vi "check convergence.vi"(4 "number of function evaluations":i32, 6 "current iteration":i32, 7 "stopping criteria":T1={"function tolerance"=1e-06, "parameter tolerance"=1e-06, "max iterations"=0, "max function calls"=0, "gradient tolerance"=0.0, "max time (sec)"=1000.0, "initial tick count"=0}, 9 "gradient":dbl[](array[numeric]), 10 "X":dbl[](array[numeric]), 11 "f":dbl) -> (0 "error out":errorcluster, 1 "xtol":dbl, 2 "ftol":dbl, 3 "stop?":bool, 5 "line search tol":dbl)   [LabVIEW 2017, in "NI_Gmath.lvlib"]
uses:
  <vilib>/gmath/NI_Gmath.lvlib
  <vilib>/gmath/NumericalOptimization/stopping criteria with time.ctl
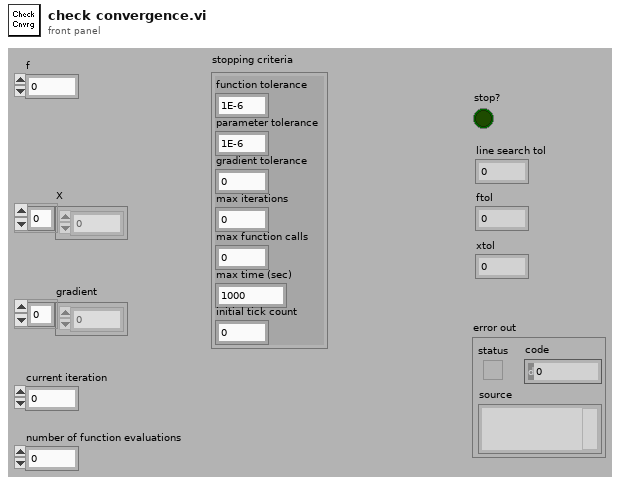
[diagram p1: front panel]
types:
  T1 = typedef "NI_Gmath.lvlib/stopping criteria with time.ctl" = cluster{"function tolerance":dbl, "parameter tolerance":dbl, "max iterations":i32, "max function calls":i32, "gradient tolerance":dbl, "max time (sec)":dbl, "initial tick count":u32}
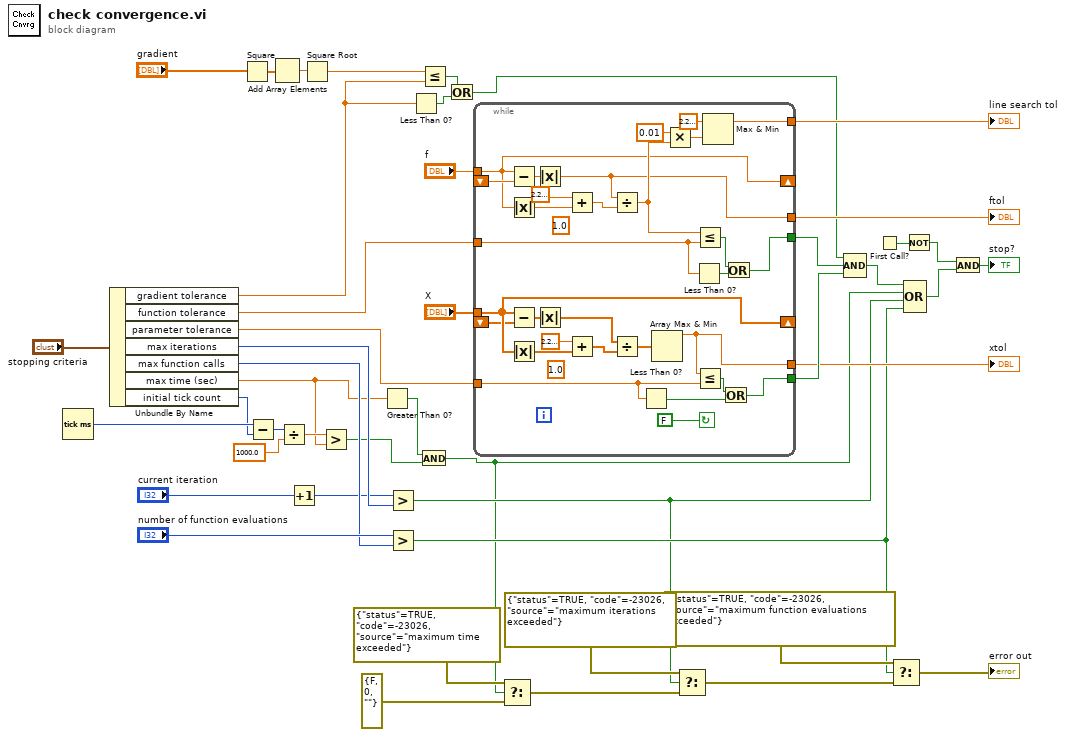
[diagram p0: block diagram]
diagram:
  n1 = Tick Count (ms)() -> (millisecond timer value=w7:u32)
  n2 = Unbundle By Name("stopping criteria") -> ("gradient tolerance"=w21:dbl, "function tolerance"=w40:dbl, "parameter tolerance"=w39:dbl, "max iterations"=w37:i32, "max function calls"=w36:i32, "max time (sec)"=w2:dbl, "initial tick count"=w6:u32)
  n3 = Square(x="gradient") -> (x^2=w25:dbl[])
  n4 = Subtract(x=w7, y=w6) -> (x-y=w5:u32)
  n5 = Add Array Elements(numeric array=w25) -> (sum=w24:dbl)
  n6 = Divide(x=w5, y=1000.0) -> (x/y=w3:dbl)
  n7 = Increment(x="current iteration") -> (x+1=w32:i32)
  n8 = Square Root(x=w24) -> (sqrt(x)=w23:dbl)
  n9 = Greater?(x=w3, y=w2) -> (0:w1:bool)
  n10 = Greater Than 0?(x=w2) -> (x > 0?=w9:bool)
  n11 = Greater?(x=w32, y=w37) -> (0:w10:bool)
  n12 = Greater?(x="number of function evaluations", y=w36) -> (0:w11:bool)
  n13 = Less Than 0?(x=w21) -> (x < 0?=w22:bool)
  n14 = And(x=w9, y=w1) -> (x .and. y?=w8:bool)
  n15 = Less Or Equal?(x=w23, y=w21) -> (x <= y?=w20:bool)
  n16 = Or(x=w20, y=w22) -> (x .or. y?=w19:bool)
  n17 = while {
    shift-right: [w67] -> _
    shift-left: _ -> [w68]
    tunnel: "f" -> [w67]
    tunnel: [w49] -> w43
    tunnel: "X" -> [w75]
    shift-right: [w75] -> _
    shift-left: _ -> [w74]
    tunnel: [w52] -> w42
    tunnel: w40 -> [w56]
    tunnel: w39 -> [w55]
    tunnel: [w58] -> w29
    tunnel: [w73] -> w28
    tunnel: [w69] -> w27
    stop <- FALSE continue-if-true
    (unwired) 1.0
    (unwired) 1.0
    n18 = Subtract(x=w67, y=w68) -> (x-y=w59:dbl)
    n19 = Absolute Value(x=w67) -> (abs(x)=w66:dbl)
    n20 = Subtract(x=w75, y=w74) -> (x-y=w60:dbl[])
    n21 = Absolute Value(x=w75) -> (abs(x)=w63:dbl[])
    n22 = Absolute Value(x=w59) -> (abs(x)=w58:dbl)
    n23 = Absolute Value(x=w60) -> (abs(x)=w57:dbl[])
    n24 = Add(x=2.220446049250313e-16 ("machine eps"), y=w66) -> (x+y=w64:dbl)
    n25 = Add(x=2.220446049250313e-16 ("machine eps"), y=w63) -> (x+y=w62:dbl[])
    n26 = Divide(x=w58, y=w64) -> (x/y=w71:dbl)
    n27 = Divide(x=w57, y=w62) -> (x/y=w61:dbl[])
    n28 = Less Than 0?(x=w55) -> (x < 0?=w54:bool)
    n29 = Array Max & Min(array=w61) -> (max value=w73:dbl)  [unwired: 3 out]
    n30 = Multiply(x=0.01, y=w71) -> (x*y=w70:dbl)
    n31 = Less Than 0?(x=w56) -> (x < 0?=w51:bool)
    n32 = Less Or Equal?(x=w71, y=w56) -> (x <= y?=w50:bool)
    n33 = Less Or Equal?(x=w73, y=w55) -> (x <= y?=w53:bool)
    n34 = Max & Min(x=2.220446049250313e-16 ("machine eps"), y=w70) -> (max(x,y)=w69:dbl)  [unwired: 1 out]
    n35 = Or(x=w53, y=w54) -> (x .or. y?=w52:bool)
    n36 = Or(x=w50, y=w51) -> (x .or. y?=w49:bool)
  }
  "ftol" <- w29
  "xtol" <- w28
  "line search tol" <- w27
  n37 = Select(t=errorcluster {"status"=TRUE, "code"=-23026, "source"="maximum time exceeded"} ("error out"), s=w8, f=errorcluster {"status"=FALSE, "code"=0, "source"=""}) -> (s? t:f=w16:errorcluster)
  n38 = Select(t=errorcluster {"status"=TRUE, "code"=-23026, "source"="maximum iterations exceeded"} ("error out"), s=w10, f=w16) -> (s? t:f=w14:errorcluster)
  n39 = Compound Arithmetic op=AND(w19, w43, w42) -> (w30:bool)
  n40 = First Call?() -> (First Call?: T/F=w35:bool)
  n41 = Select(t=errorcluster {"status"=TRUE, "code"=-23026, "source"="maximum function evaluations exceeded"} ("error out"), s=w11, f=w14) -> (s? t:f=→"error out":errorcluster)
  n42 = Not(x=w35) -> (.not. x?=w33:bool)
  n43 = Compound Arithmetic op=OR(w30, w8, w10, w11) -> (w31:bool)
  n44 = And(x=w33, y=w31) -> (x .and. y?=→"stop?":bool)
